vi "Excel Find and Replace.vi"   [LabVIEW 2010, in "NI_ReportGenerationToolkit.lvlib"]
doc: "Searches the occurrences of <B>searched string</B> and replaces them with a new string or numeric value. The data type you wire to the <B>replacement</B> input determines the polymorphic instance to use."
uses:
  <vilib>/addons/_office/NI_ReportGenerationToolkit.lvlib
  <vilib>/Utility/NIReport.llb/Excel/NI_Excel.lvclass
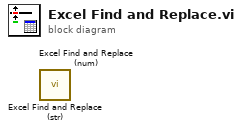
[diagram p0: block diagram]
diagram:
  n1 = call <vilib>:"Excel Find and Replace (str).vi"() -> ()  [unwired: 13 in, 3 out]
  n2 = call "Excel Find and Replace (num).vi"() -> ()  [unwired: 13 in, 3 out]
